vi "skip latter choose step.vi"(7 "step number":i32, 8 "error In":errorcluster, 9 "JSON string":string, 10 "Step order":string, 11 "process_ID":string) -> (0 "error IO":errorcluster, 5 "step number after":i32)   [LabVIEW 2020]
uses:
  status/skip_latter.vi
  status/skip_status.vi
  status/emergency stop.vi
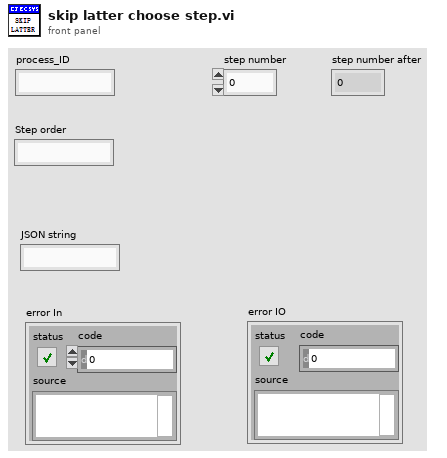
[diagram p1: front panel]
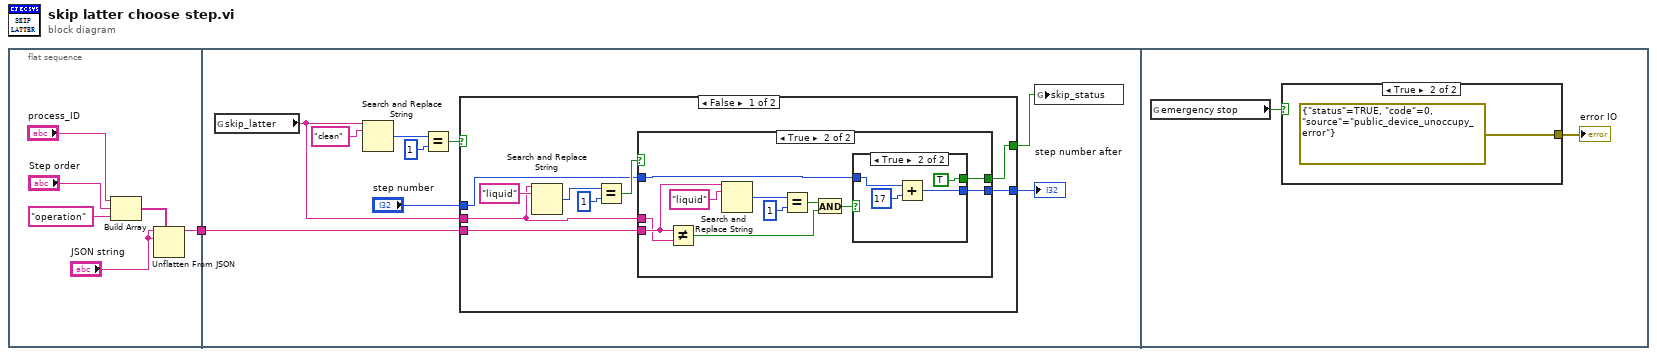
[diagram p0: block diagram]
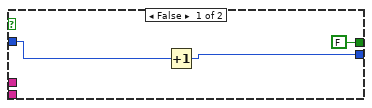
[diagram p2: hidden frame]
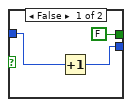
[diagram p3: hidden frame]
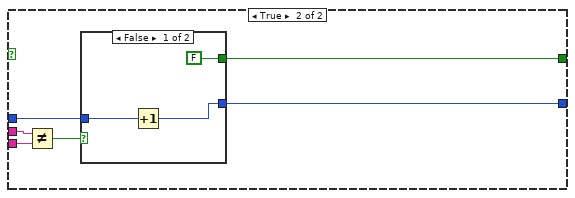
[diagram p4: hidden frame]
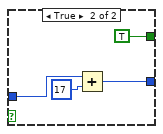
[diagram p5: hidden frame]
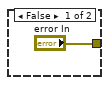
[diagram p6: hidden frame]
diagram:
  n1 = flat-sequence {
    tunnel: [w2] -> w1
    tunnel: w1 -> [w11]
    frame #0 {
      n2 = Build Array("process_ID", "Step order", "operation" ("string")) -> (w6:string[])
      n3 = Unflatten From JSON(path=w6, JSON string="JSON string", type and defaults="JSON string") -> (value=w2:string)  [unwired: 4 in, 1 out]
    }
    frame #1 {
      n4 = global read "skip_latter.vi" "skip_latter"() -> (w12:string)
      n5 = Search and Replace String(input string=w12, search string="clean") -> (number of replacements=w16:i32)  [unwired: 6 in, 3 out]
      n6 = Equal?(x=w16, y=1) -> (x = y?=w13:bool)
      n7 = case shown="False" w13 {
        tunnel: w12 -> [w20 w51]
        tunnel: w11 -> [w21 w50]
        tunnel: "step number" -> [w17 w49]
        tunnel: [w18 w48] -> w9
        tunnel: [w19 w47] -> w8
        frame False {
          n8 = Search and Replace String(input string=w20, search string="liquid") -> (number of replacements=w25:i32)  [unwired: 6 in, 3 out]
          n9 = Equal?(x=w25, y=1) -> (x = y?=w22:bool)
          n10 = case shown="True" w22 {
            tunnel: w21 -> [_ w34]
            tunnel: w20 -> [_ w33]
            tunnel: [FALSE ("skip_status") w31] -> w19
            tunnel: [w27 w30] -> w18
            tunnel: w17 -> [w28 w29]
            frame False {
              n11 = Increment(x=w28) -> (x+1=w27:i32)
            }
            frame True {
              n12 = Not Equal?(x=w34, y=w33) -> (x != y?=w35:bool)
              n13 = Search and Replace String(input string=w34, search string="liquid") -> (number of replacements=w39:i32)  [unwired: 6 in, 3 out]
              n14 = Equal?(x=w39, y=1) -> (x = y?=w36:bool)
              n15 = And(x=w36, y=w35) -> (x .and. y?=w32:bool)
              n16 = case shown="True" w32 {
                tunnel: [FALSE ("skip_status") TRUE ("skip_status")] -> w31
                tunnel: [w41 w44] -> w30
                tunnel: w29 -> [w40 w43]
                frame False {
                  n17 = Increment(x=w40) -> (x+1=w41:i32)
                }
                frame True {
                  n18 = Add(x=w43, y=17) -> (x+y=w44:i32)
                }
              }
            }
          }
        }
        frame True {
          n19 = Not Equal?(x=w51, y=w50) -> (x != y?=w52:bool)
          n20 = case shown="False" w52 {
            tunnel: w49 -> [w55 w58]
            tunnel: [w54 w57] -> w48
            tunnel: [FALSE ("skip_status") TRUE ("skip_status")] -> w47
            frame False {
              n21 = Increment(x=w55) -> (x+1=w54:i32)
            }
            frame True {
              n22 = Add(x=w58, y=17) -> (x+y=w57:i32)
            }
          }
        }
      }
      "step number after" <- w9
      n23 = global write "skip_status.vi" "skip_status"(w8) -> ()
    }
    frame #2 {
      n24 = global read "emergency stop.vi" "emergency stop"() -> (w60:bool)
      n25 = case shown="True" w60 {
        tunnel: ["error In" errorcluster {"status"=TRUE, "code"=0, "source"="public_device_unoccupy_error"} ("error IO")] -> w61
        frame False {
        }
        frame True {
        }
      }
      "error IO" <- w61
    }
  }
